vi "Execute.vi"(5 "Init user event out":refnum<user-event>, 7 "user event in":refnum<user-event>, 8 "Advanced Waveform In":refnum<class "Advanced Waveform.lvclass">, 9 "Generate Signal Message in":refnum<class "Generate Signal Message.lvclass">, 10 "Command Queue":refnum<queue>, 11 "error in (no error)":errorcluster) -> (0 "Advanced Waveform Out":refnum<class "Advanced Waveform.lvclass">, 1 "Generate Signal Message out":refnum<class "Generate Signal Message.lvclass">, 2 "Stop":bool, 3 "error out":errorcluster)   [LabVIEW 2011, in "Generate Signal Message.lvclass"]
uses:
  Generate Signal Message.lvclass
  Advanced Waveform Class/Advanced Waveform.lvclass
  Message.lvclass
  Display Message/Display Message.lvclass
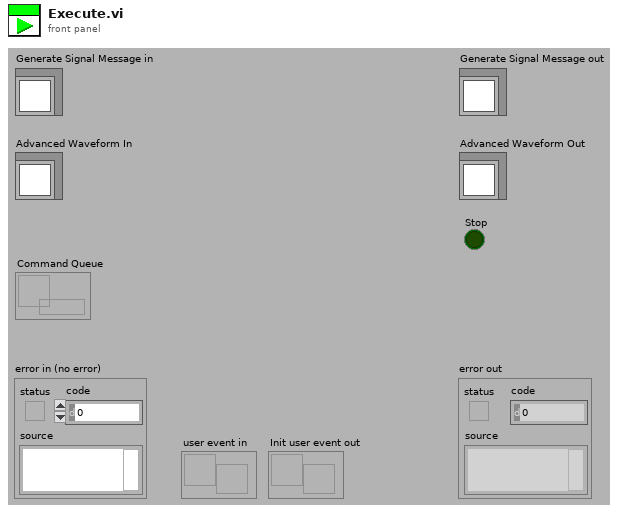
[diagram p1: front panel]
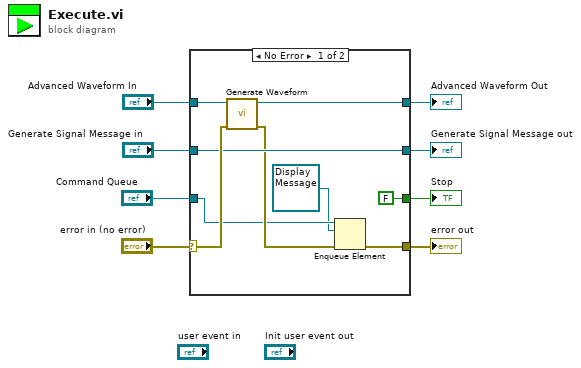
[diagram p0: block diagram]
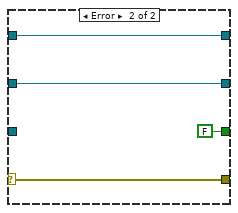
[diagram p2: hidden frame]
diagram:
  n1 = case shown="No Error" "error in (no error)" {
    selector: "error in (no error)" -> [w15 w19]
    tunnel: "Advanced Waveform In" -> [w17 w21]
    tunnel: [w16 w21] -> w6
    tunnel: [w11 w19] -> w5
    tunnel: [w14 w20] -> w4
    tunnel: "Generate Signal Message in" -> [w14 w20]
    tunnel: [FALSE FALSE] -> w2
    tunnel: "Command Queue" -> [w10 _]
    frame No Error {
      n2 = call-dynamic "Generate Waveform.vi"("error in (no error)"=w15, "Waveform in"=w17) -> ("error out"=w12:errorcluster, "Waveform out"=w16:refnum<class "Advanced Waveform.lvclass">)  [unwired: 8 in]
      n3 = Enqueue Element(queue=w10, element=refnum<class "Display Message.lvclass"> refnum ("Display Message.lvclass"), error in (no error)=w12) -> (error out=w11:errorcluster)  [unwired: 1 in, 2 out]
    }
    frame Error {
    }
  }
  "error out" <- w5
  "Generate Signal Message out" <- w4
  "Stop" <- w2
  "Advanced Waveform Out" <- w6
